vi "Read Handle.vi"(8 "error in (no error)":errorcluster, 11 "HandleHolder in":refnum<class "HandleHolder.lvclass">) -> (0 "error out":errorcluster, 2 "Handle":refnum<class "LoggingHandle.lvclass">, 3 "HandleHolder out":refnum<class "HandleHolder.lvclass">)   [LabVIEW 2024, in "HandleHolder.lvclass"]
uses:
  HandleHolder.lvclass
  LogHandle/Interface/LoggingHandle.lvclass
  HandleHolder.lvclass/HandleHolder.ctl
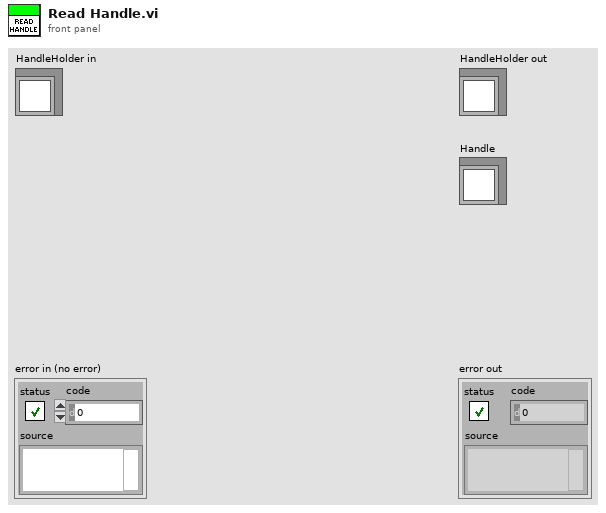
[diagram p1: front panel]
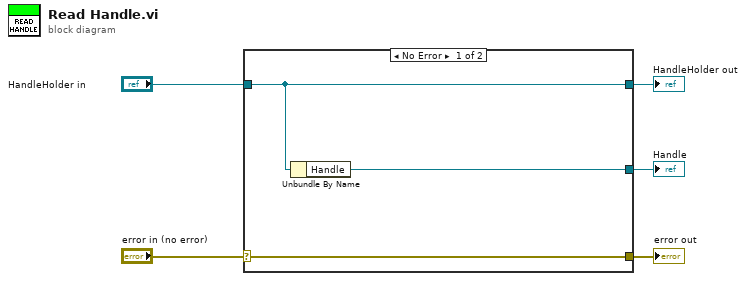
[diagram p0: block diagram]
diagram:
  n1 = case shown="No Error" "error in (no error)" {
    selector: "error in (no error)" -> [w8 w9]
    tunnel: [w8 w9] -> w4
    tunnel: [w7 w10] -> w2
    tunnel: "HandleHolder in" -> [w7 w10]
    tunnel: [w6 _] -> w1
    frame No Error {
      n2 = Unbundle By Name(w7) -> ("Handle"=w6:refnum<class "LoggingHandle.lvclass">)
    }
    frame Error {
    }
  }
  "error out" <- w4
  "HandleHolder out" <- w2
  "Handle" <- w1
